vi "C4Ftr_getType.vi"(0 "c4Ftr in":refnum<k24>, 11 "error in":errorcluster) -> (4 "c4Ftr out":refnum<k24>, 6 "type out":i64(ring) items=["UNKNOWN", "INTEGER", "FLOAT", "STRING", "ENUMERATION", "COMMAND", "BOOLEAN"], 15 "error out":errorcluster)   [LabVIEW 2015, in "libC4HdlLV.lvlib"]
uses:
  libC4HdlLV.lvlib
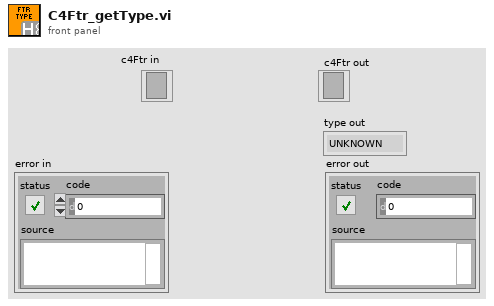
[diagram p1: front panel]
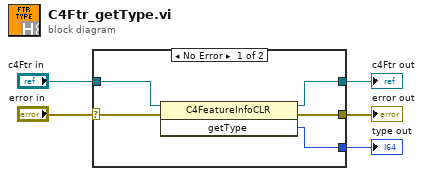
[diagram p0: block diagram]
diagram:
  n1 = case shown="No Error" "error in" {
    selector: "error in" -> [w10 w12]
    tunnel: "c4Ftr in" -> [w9 w11]
    tunnel: [w8 _] -> w3
    tunnel: [w7 w12] -> w2
    tunnel: [w6 w11] -> w1
    frame No Error {
      n2 = invoke class="C4FeatureInfoCLR" method="getType"(reference=w9, error in=w10) -> (reference out=w6:refnum<k24>, error out=w7:errorcluster, "getType"=w8:i64)  [unwired: 1 in]
    }
    frame Error {
    }
  }
  "error out" <- w2
  "type out" <- w3
  "c4Ftr out" <- w1
